vi "ColorIndicators_2Colors.vi"(6 "Numeric":dbl, 9 "alarm 1":dbl, 10 "alarm 2":dbl, 11 "Digital in":refnum<vi>) -> ()   [LabVIEW 2016]
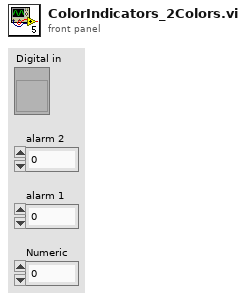
[diagram p1: front panel]
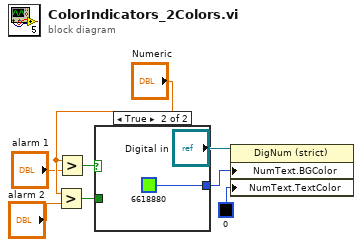
[diagram p0: block diagram]
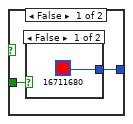
[diagram p2: hidden frame]
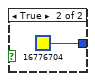
[diagram p3: hidden frame]
diagram:
  n1 = Greater?(x="Numeric", y="alarm 2") -> (0:w5:bool)
  n2 = Greater?(x="Numeric", y="alarm 1") -> (0:w2:bool)
  n3 = case shown="True" w2 {
    tunnel: [w9 u32 6618880] -> w7
    tunnel: w5 -> [w10 _]
    frame False {
      n4 = case shown="False" w10 {
        tunnel: [u32 16711680 u32 16776704] -> w9
        frame False {
        }
        frame True {
        }
      }
    }
    frame True {
    }
  }
  n5 = property on="Property Node" class="DigNum (strict)"(reference="Digital in", "NumText.BGColor"=w7, "NumText.TextColor"=u32 0) -> ()  [unwired: 1 in, 2 out]
